vi "Agilent34410A Get TrigSource.vi"(8 "error in (no error)":errorcluster, 11 "VISA Rsrc":refnum<visa-resource-name>="SR530") -> (0 "error out":errorcluster, 1 "TrigSrc String":string, 2 "Trigger Source":enum16{"Immediate", "External", "Bus"}(ring), 3 "VISA Rsrc Out":refnum<visa-resource-name>="GPIB0::12::INSTR", 4 "ChaineRep":string caption="Chaîne de commande")   [LabVIEW 2019]
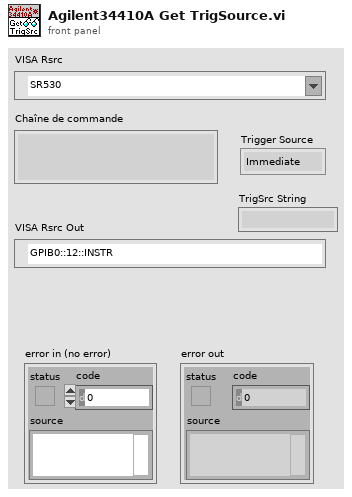
[diagram p1: front panel]
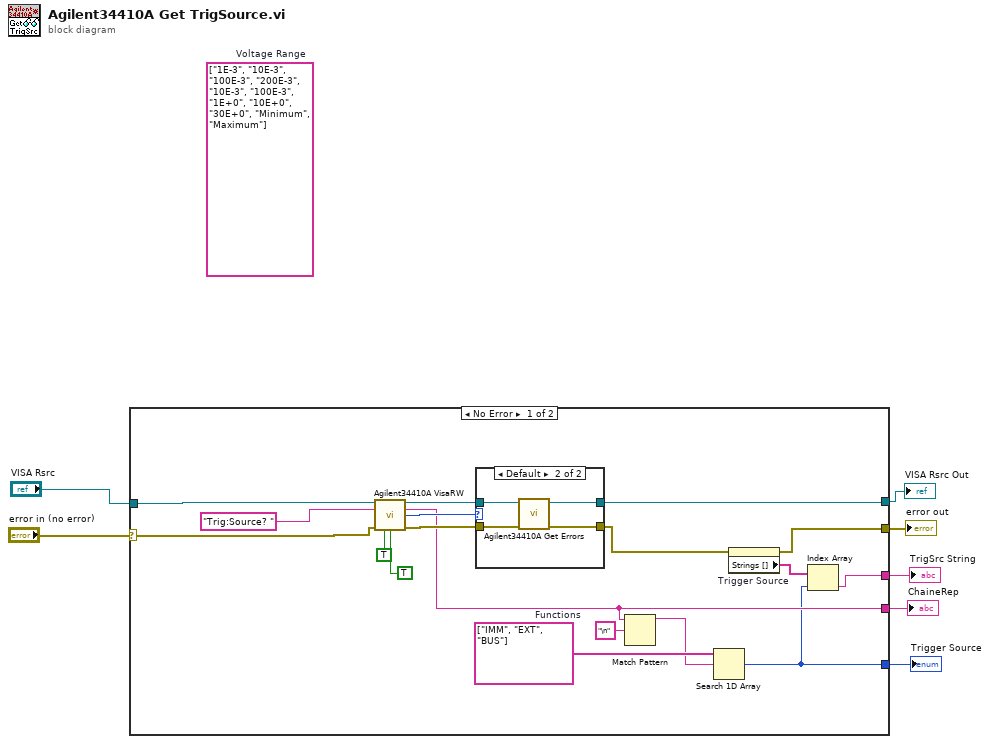
[diagram p0: block diagram]
diagram:
  (unwired) string[] ["1E-3", "10E-3", "100E-3", "200E-3", "10E-3", "100E-3", "1E+0", "10E+0", "30E+0", "Minimum", "Maximum"]  # Voltage Range
  n1 = case shown="No Error" "error in (no error)" {
    selector: "error in (no error)" -> [w18 w32]
    tunnel: "VISA Rsrc" -> [w25 w33]
    tunnel: [w11 w32] -> w5
    tunnel: [w24 w33] -> w4
    tunnel: [w15 _] -> w3
    tunnel: [w9 _] -> w2
    tunnel: [w8 _] -> w1
    frame No Error {
      w16 = string[] ["IMM", "EXT", "BUS"]  # Functions
      n2 = call <userlib>:"Agilent34410A VisaRW.vi"("VISA Rsrc"=w25, "ChaineCom"="Trig:Source? " ("string (\"\")"), "error in (no error)"=w18, "Lecture?(T)"=TRUE, "Poll?(F)"=TRUE) -> ("VISA Rsrc Out"=w22:refnum<visa-resource-name>, "ChaineRep"=w15:string, "octet d'état"=w21:u16, "error out"=w20:errorcluster)  [unwired: 6 in, 1 out]
      n3 = case shown="Default" w21 {
        tunnel: w22 -> [w27 w31]
        tunnel: w20 -> [w26 w30]
        tunnel: [w26 w29] -> w12
        tunnel: [w27 w28] -> w24
        frame 0 {
        }
        frame Default {
          n4 = call <userlib>:"Agilent34410A Get Errors.vi"("error in (no error)"=w30, "VISA Rsrc"=w31) -> ("error out"=w29:errorcluster, "VISA Rsrc Out"=w28:refnum<visa-resource-name>)  [unwired: 7 in, 1 out]
        }
      }
      n5 = Match Pattern(string=w15, regular expression="\n" ("expression régulière")) -> (before substring=w13:string)  [unwired: 1 in, 3 out]
      n6 = Search 1D Array(1D array=w16, element=w13) -> (index of element=w9:i32)  [unwired: 1 in]
      n7 = property on="Trigger Source" class="Énum (strict)"(error in=w12) -> (error out=w11:errorcluster, "Strings []"=w10:string[])  [unwired: 1 in, 1 out]
      n8 = Index Array(array=w10, index=w9) -> (element=w8:string)
    }
    frame Error {
    }
  }
  "error out" <- w5
  "VISA Rsrc Out" <- w4
  "ChaineRep" <- w3
  "Trigger Source" <- w2
  "TrigSrc String" <- w1
